vi "MDOIncorporate New Data.vi"(8 "error in (no error)":errorcluster, 9 "New Current Data":waveform(dbl), 10 "New Voltage Data":waveform(dbl), 11 "Data in":T1={"UI References"={"Stop Ref"=refnum, "Save Ref"=refnum, "Open Ref"=refnum, "Export Ref"=refnum, "Acquire Ref"=refnum, "Configure Ref"=refnum, "Clear Ref"=refnum, "Analyze Ref"=refnum, "Status Ref"=refnum, "Snapshot Ref"=refnum, "Cancel"=refnum, "Graph Ref"=refnum}, "Graph Data"={"Voltage Data"=[], "Annotation List"=[], "Cursor List"=[], "Voltage Analysis Data"=[], "Current Data"=[], "Current Analysis Data"=[]}, "User Specified"={"Hardware Configuration"={"SyncMode"=0, "Current_FIR_filter"=FALSE}, "New Data Behavior"=enum."Replace", "Acquire Type"=enum."Triggered", "Data_save_directory"=path ""}, "Coeff"={"Coeff_U"=300.0, "Offset_U"=0.0, "Coeff_I"=23.5, "Offset_I"=0.15}} {"User Specified"."Hardware Configuration"."SyncMode" items=["INTERNAL"=0, "EXTERNAL_MASTER"=1, "DI_SYN1_RISE"=2, "DI_SYN1_FALL"=3, "DI_SYN2_RISE"=6, "DI_SYN2_FALL"=7]}) -> (0 "error out":errorcluster, 3 "Data out":T1={"UI References"={"Stop Ref"=refnum, "Save Ref"=refnum, "Open Ref"=refnum, "Export Ref"=refnum, "Acquire Ref"=refnum, "Configure Ref"=refnum, "Clear Ref"=refnum, "Analyze Ref"=refnum, "Status Ref"=refnum, "Snapshot Ref"=refnum, "Cancel"=refnum, "Graph Ref"=refnum}, "Graph Data"={"Voltage Data"=[], "Annotation List"=[], "Cursor List"=[], "Voltage Analysis Data"=[], "Current Data"=[], "Current Analysis Data"=[]}, "User Specified"={"Hardware Configuration"={"SyncMode"=0, "Current_FIR_filter"=FALSE}, "New Data Behavior"=enum."Replace", "Acquire Type"=enum."Triggered", "Data_save_directory"=path ""}, "Coeff"={"Coeff_U"=300.0, "Offset_U"=0.0, "Coeff_I"=23.5, "Offset_I"=0.15}} {"User Specified"."Hardware Configuration"."SyncMode" items=["INTERNAL"=0, "EXTERNAL_MASTER"=1, "DI_SYN1_RISE"=2, "DI_SYN1_FALL"=3, "DI_SYN2_RISE"=6, "DI_SYN2_FALL"=7]})   [LabVIEW 2012]
doc: "Incorporates newly acquired or loaded data into the main state data. New data can replace, be appended to, or overlayed over (as an additional channel) existing data. If the user does not have a preference saved a dialog will be presented asking which method to use."
uses:
  controls/MDOData.ctl
  controls/MDOUI References.ctl
  controls/MDOGraph Data.ctl
  <vilib>/Utility/miscctls.llb/LVAnnotationListTypeDef.ctl
  <vilib>/Utility/miscctls.llb/LVCursorListTypeDef.ctl
  controls/MDOUser Specified Data.ctl
  controls/MDOHW Configuration.ctl
  controls/MDONew Data Behavior.ctl
  controls/Acquire_Type.ctl
  controls/Coeff.ctl
panel:
  # "(Scroll up to see large state data in/out clusters)"
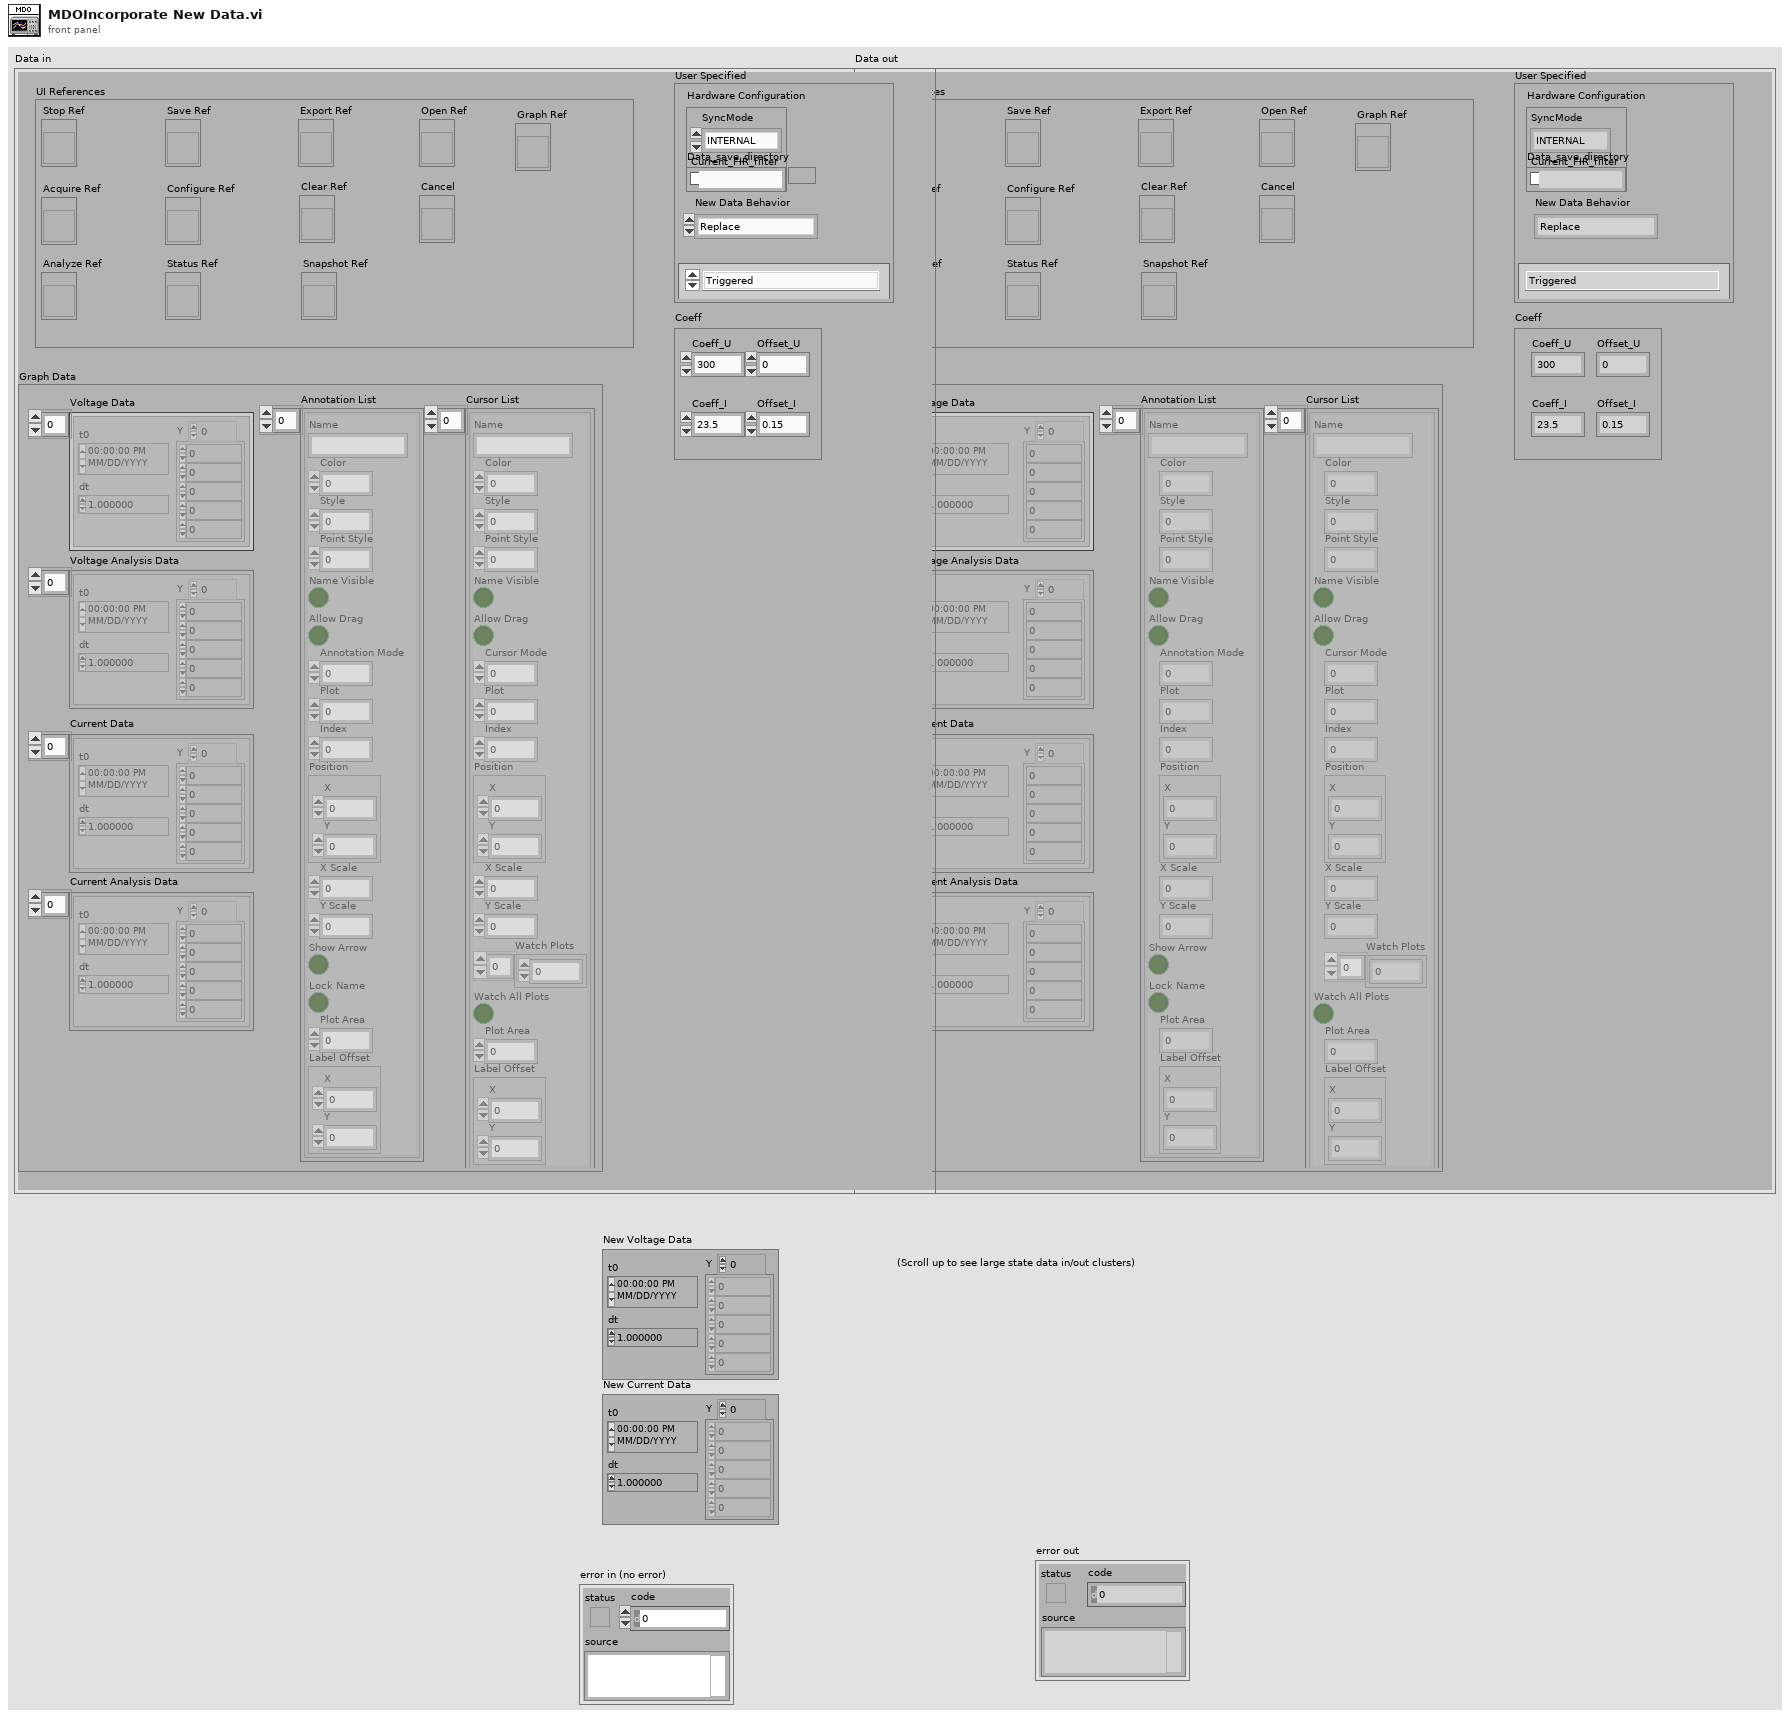
[diagram p1: front panel]
types:
  T1 = typedef "MDOData.ctl" = cluster{"UI References":T2, "Graph Data":T3, "User Specified":T6, "Coeff":T10}
  T2 = typedef "MDOUI References.ctl" = cluster{"Stop Ref":refnum<vi>, "Save Ref":refnum<vi>, "Open Ref":refnum<vi>, "Export Ref":refnum<vi>, "Acquire Ref":refnum<vi>, "Configure Ref":refnum<vi>, "Clear Ref":refnum<vi>, "Analyze Ref":refnum<vi>, "Status Ref":refnum<vi>, "Snapshot Ref":refnum<vi>, "Cancel":refnum<vi>, "Graph Ref":refnum<vi>}
  T3 = typedef "MDOGraph Data.ctl" = cluster{"Voltage Data":waveform(dbl)[], "Annotation List":T4, "Cursor List":T5, "Voltage Analysis Data":waveform(dbl)[], "Current Data":waveform(dbl)[], "Current Analysis Data":waveform(dbl)[]}
  T4 = typedef "LVAnnotationListTypeDef.ctl" = cluster{"Name":string, "Color":u32, "Style":u8, "Point Style":u8, "Name Visible":bool, "Allow Drag":bool, "Annotation Mode":u32, "Plot":i32, "Index":i32, "Position":cluster{"X":dbl, "Y":dbl}, "X Scale":u32, "Y Scale":u32, "Show Arrow":bool, "Lock Name":bool, "Plot Area":i32, "Label Offset":cluster{"X":dbl, "Y":dbl}}[]
  T5 = typedef "LVCursorListTypeDef.ctl" = cluster{"Name":string, "Color":u32, "Style":u8, "Point Style":u8, "Name Visible":bool, "Allow Drag":bool, "Cursor Mode":u32, "Plot":i32, "Index":i32, "Position":cluster{"X":dbl, "Y":dbl}, "X Scale":u32, "Y Scale":u32, "Watch Plots":i32[], "Watch All Plots":bool, "Plot Area":i32, "Label Offset":cluster{"X":dbl, "Y":dbl}}[]
  T6 = typedef "MDOUser Specified Data.ctl" = cluster{"Hardware Configuration":T7, "New Data Behavior":T8, "Acquire Type":T9, "Data_save_directory":path}
  T7 = typedef "MDOHW Configuration.ctl" = cluster{"SyncMode":u32, "Current_FIR_filter":bool}
  T8 = typedef "MDONew Data Behavior.ctl" = enum16{"Replace", "Overlay", "Append"}
  T9 = typedef "Acquire_Type.ctl" = enum16{"Triggered", "Continues"}
  T10 = typedef "Coeff.ctl" = cluster{"Coeff_U":dbl, "Offset_U":dbl, "Coeff_I":dbl, "Offset_I":dbl}
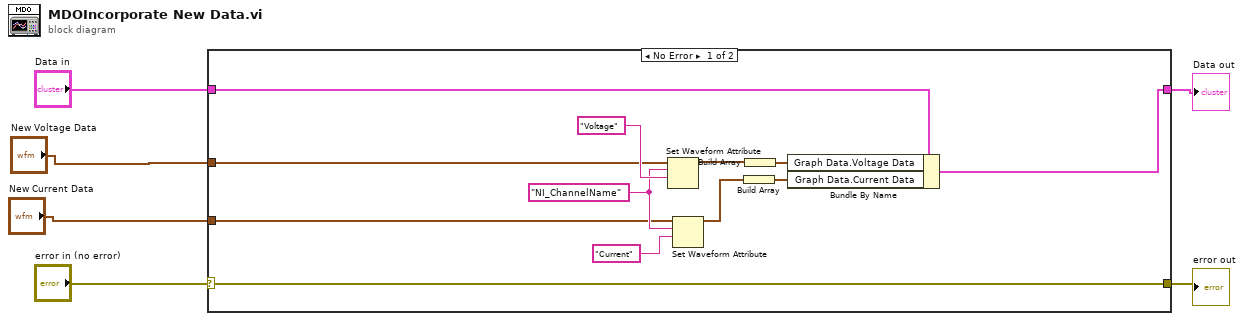
[diagram p0: block diagram]
diagram:
  n1 = case shown="No Error" "error in (no error)" {
    selector: "error in (no error)" -> [w16 w20]
    tunnel: "Data in" -> [w18 w19]
    tunnel: "New Voltage Data" -> [w8 _]
    tunnel: [w17 w19] -> w5
    tunnel: [w16 w20] -> w3
    tunnel: "New Current Data" -> [w7 _]
    frame No Error {
      w10 = "NI_ChannelName" ("name")
      n2 = Set Waveform Attribute(5:"Voltage" ("name"), 6:w10, 7:w8) -> (3:w13:waveform(dbl))  [unwired: 1 in, 2 out]
      n3 = Set Waveform Attribute(5:"Current" ("name"), 6:w10, 7:w7) -> (3:w12:waveform(dbl))  [unwired: 1 in, 2 out]
      n4 = Build Array(w12) -> (w14:waveform(dbl)[])
      n5 = Build Array(w13) -> (w15:waveform(dbl)[])
      n6 = Bundle By Name(cluster=w18, "Graph Data.Voltage Data"=w15, "Graph Data.Current Data"=w14) -> (w17:T1)
    }
    frame Error {
    }
  }
  "Data out" <- w5
  "error out" <- w3
